vi "TestRingdownEvent.vi"() -> ()   [LabVIEW 2014, in "EventModule.lvlib"]
uses:
  EventModule.lvlib
  EventPlugins/EventPluginBaseClass/TypeDefs/clEvtConfig.ctl
  PublicAPI/Arguments/Requests/dblEvtParams.ctl
  PublicAPI/Arguments/Requests/dblTimeArray.ctl
  EventPlugins/EventPluginBaseClass/TypeDefs/clEvtReportArray.ctl
  EventPlugins/EventPluginBaseClass/TypeDefs/clEvtReport.ctl
  EventPlugins/EventPluginBaseClass/TypeDefs/dblEvtSignalArray.ctl
  TestInfo.ctl
  <userlib>/NIST/ModuleAdminLib/ModuleAdmin/ModuleAdmin.lvclass
  PublicAPI/Arguments/Broadcasts/clDidInit.ctl
  <userlib>/NIST/ModuleAdminLib/ModuleAdmin/ModuleAdmin.lvclass/ModuleAdmin.ctl
  PublicAPI/Arguments/Requests/clStopArgument.ctl
  PublicAPI/Arguments/Broadcasts/clStatUpdate.ctl
  PublicAPI/Arguments/Broadcasts/clErrorRpt.ctl
  <userlib>/NIST/ModuleAdminLib/ModuleAdmin/Accessors/Read CloneRegRef.vi
  <vilib>/Analysis/1siggen.llb/Ramp Pattern by Delta.vi
  <userlib>/NIST/ModuleAdminLib/CloneRegistration/CloneRegistration.lvclass
  EventPlugins/EventPluginBaseClass/EventPluginBaseClass.lvclass
  <vilib>/Analysis/NI_AALBase.lvlib
panel:
  in  "End Time":dbl=10.0
  in  "Start Time":dbl
  in  "Plugin Type":u16(ring)=3 items=["C37.118.1", "Event From CSV", "IEEEBusSystem", "Ringdown", "60255Harm", "User1", "User2"]
  in  "btnGetEvtSignal":bool
  out "dblEventSignalArray":T1
  out "PathToPluginIniFileReport":path=path "P:/Framework/Events/EventPlugins/SSEvtPlugin/SteadyStateEventPlugin.ini"
  in  "btnReadPathToPlugin":bool
  in  "btnGetEvtReportArray":bool
  out "clEvtReportArray":T2 {"Synx" format="%#_4g"}
  in  "btnReadEvtParams":bool
  in  "btnWriteEvtParams":bool
  in  "btnReadTimeArray":bool
  in  "btnWriteTimeArray":bool
  out "dblTimeArrayReport":T4
  out "dblEvtParamsReport":T5
  out "dblTimeArray":T4=[0.0, 0.05, 0.1, 0.15000000000000002, 0.2]
  in  "dblEvtParams":T5=[[0.0, 0.34657, 0.69677, 1.297, 1.4569, 6.0606, 7.2288, 8.9506, 11.705, 18.574], [1000.0, 24.879, 55.751, 46.204, 36.867, 1.995, 0.82578, 1.5487, 1.8652, 1.6268], [0.0, 1.876, 0.28983, 1.5993, 2.6728, 3.9286, 1.2558, 3.3379, 3.6506, 7.1708], [0.0, -67.696, -60.912, 99.138, -123.76, 176.38, -149.46, -106.27, -18.535, -59.29], [0.0, 0.0, 0.58767, 0.6985, 1.3263, 2.7275, 7.1783, 8.122, 14.704, 15.622], [200.0, 31.231, 41.605, 48.38, 1.6511, 0.84175, 2.671, 0.64619, 0.78365, 0.6061], [0.0, 6.2405, 2.3071, 0.28998, 1.025, 3.6069, 15.284, 3.3041, 2.4034, 2.5242], [0.0, 180.0, 37.683, 113.63, 41.526, 4.7072, 5.0124, -177.41, -50.759, 41.697], [568.0, 0.0, 0.0, 0.0, 0.0, 0.0, 0.0, 0.0, 0.0, 0.0], [0.0, 0.0, 0.0, 0.0, 0.0, 0.0, 0.0, 0.0, 0.0, 0.0], [0.0, 0.0, 0.0, 0.0, 0.0, 0.0, 0.0, 0.0, 0.0, 0.0], [0.0, 0.0, 0.0, 0.0, 0.0, 0.0, 0.0, 0.0, 0.0, 0.0], [0.0, 0.0, 0.0, 0.0, 0.0, 0.0, 0.0, 0.0, 0.0, 0.0]]
  out "clEvtConfigReport":T6={"T0(UTC)"=0.0, "F0"=0.0, "Fs"=60, "FSamp"=0, "bPosSeq"=FALSE}
  in  "btnReadEvtConfig":bool
  in  "clEvtConfig":T6={"T0(UTC)"=0.0, "F0"=60.0, "Fs"=60, "FSamp"=960, "bPosSeq"=FALSE}
  in  "btnWriteEvtConfig":bool
  in  "btnLoadPlugin":bool
  in  "btnRemove":bool
  out "Status Log":string
  out "Active Modules (Array)":string[](array[string])
  in  "btnAdd":bool
  in  "btnStop":bool
  in  "Select Module":i32(ring)=-1 caption="Select Module to send Request" items=["All"=-1, "4140002"=4140002]
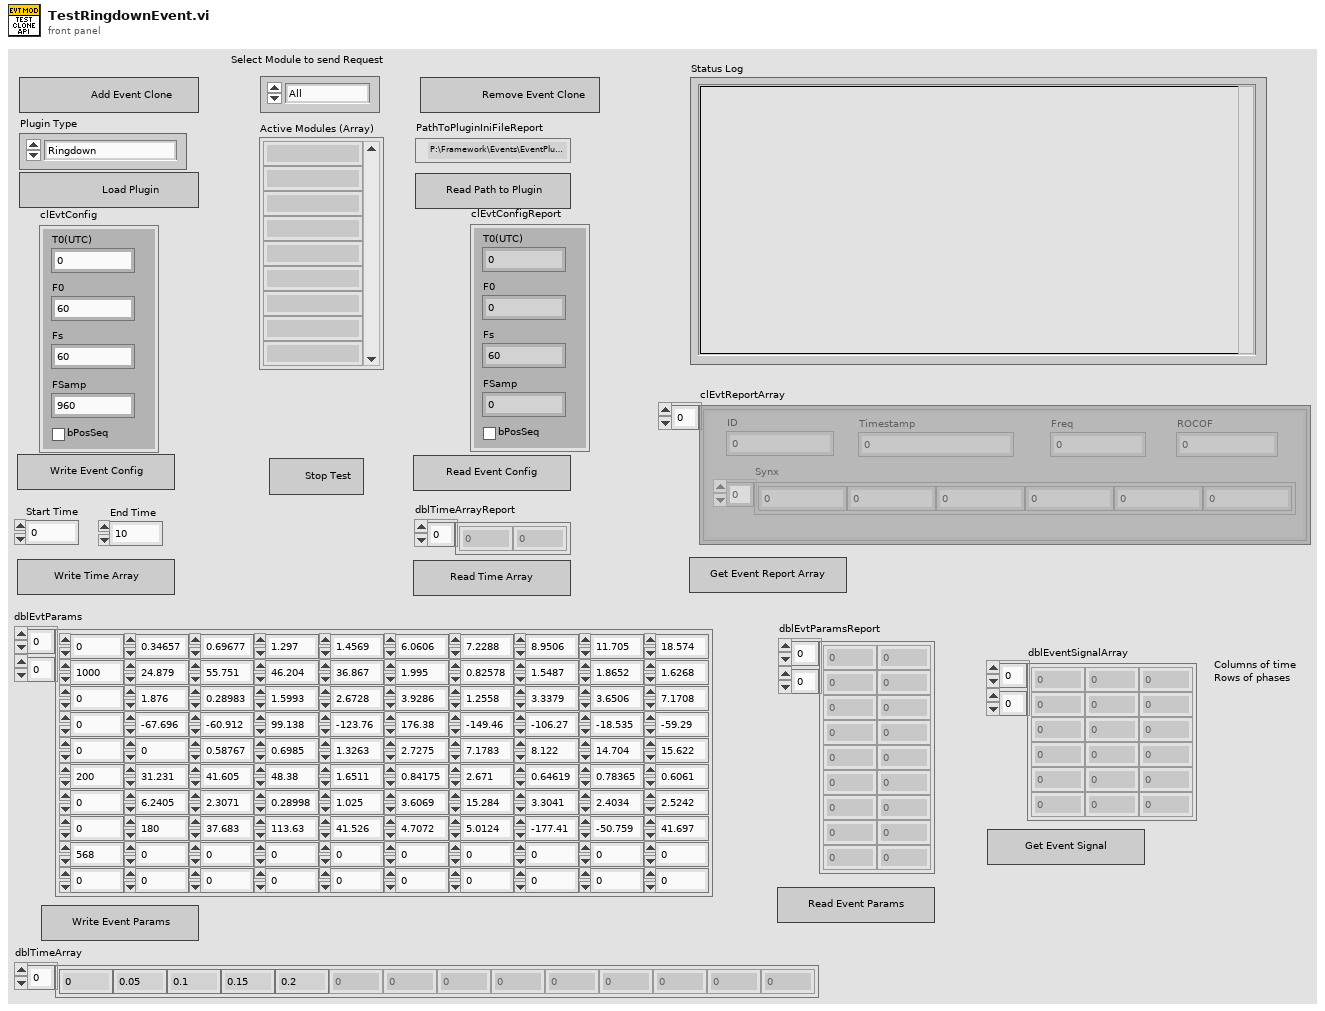
[diagram p1: front panel]
types:
  T1 = typedef "EventPlugins.lvlib/EventPluginBaseClass.lvclass/dblEvtSignalArray.ctl" = dbl[][]
  T2 = typedef "EventPlugins.lvlib/EventPluginBaseClass.lvclass/clEvtReportArray.ctl" = T3[]
  T3 = typedef "EventPlugins.lvlib/EventPluginBaseClass.lvclass/clEvtReport.ctl" = cluster{"Timestamp":dbl, "Synx":cdb[], "Freq":dbl, "ROCOF":dbl, "ID":i16}
  T4 = typedef "EventModule.lvlib/dblTimeArray.ctl" = dbl[]
  T5 = typedef "EventModule.lvlib/dblEvtParams.ctl" = dbl[][]
  T6 = typedef "EventPlugins.lvlib/EventPluginBaseClass.lvclass/clEvtConfig.ctl" = cluster{"T0(UTC)":dbl, "F0":dbl, "Fs":i32, "FSamp":u32, "bPosSeq":bool}
  T7 = typedef "EventModule.lvlib/TestInfo.ctl" = cluster{"PluginIniFilePaths":path[]}
  T8 = typedef "EventModule.lvlib/clBroadcastEvents.ctl" = cluster{"DidInit":refnum<user-event>, "StatusUpdate":refnum<user-event>, "ErrorReport":refnum<user-event>, "DidStop":refnum<user-event>, "ReadEvtConfig":refnum<user-event>, "ReadTimeArray":refnum<user-event>, "ReadEvtParams":refnum<user-event>, "GetEvtReportArray":refnum<user-event>, "ReadPathToPlugin":refnum<user-event>, "GetEvtSignal":refnum<user-event>, "ReadBusNumber":refnum<user-event>}
  T9 = typedef "EventModule.lvlib/clDidInit.ctl" = cluster{"Init?":bool, "ModuleAdmin":refnum<class "ModuleAdmin.lvclass">}
  T10 = typedef "EventModule.lvlib/clStopArgument.ctl" = cluster{"Exit via Stop Module Req?":bool, "Wait for Module to stop?":bool, "ModuleAdmin":refnum<class "ModuleAdmin.lvclass">}
  T11 = typedef "EventModule.lvlib/clStatUpdate.ctl" = cluster{"Status":string}
  T12 = typedef "EventModule.lvlib/clErrorRpt.ctl" = cluster{"error":errorcluster, "AdditionalInfo":string}
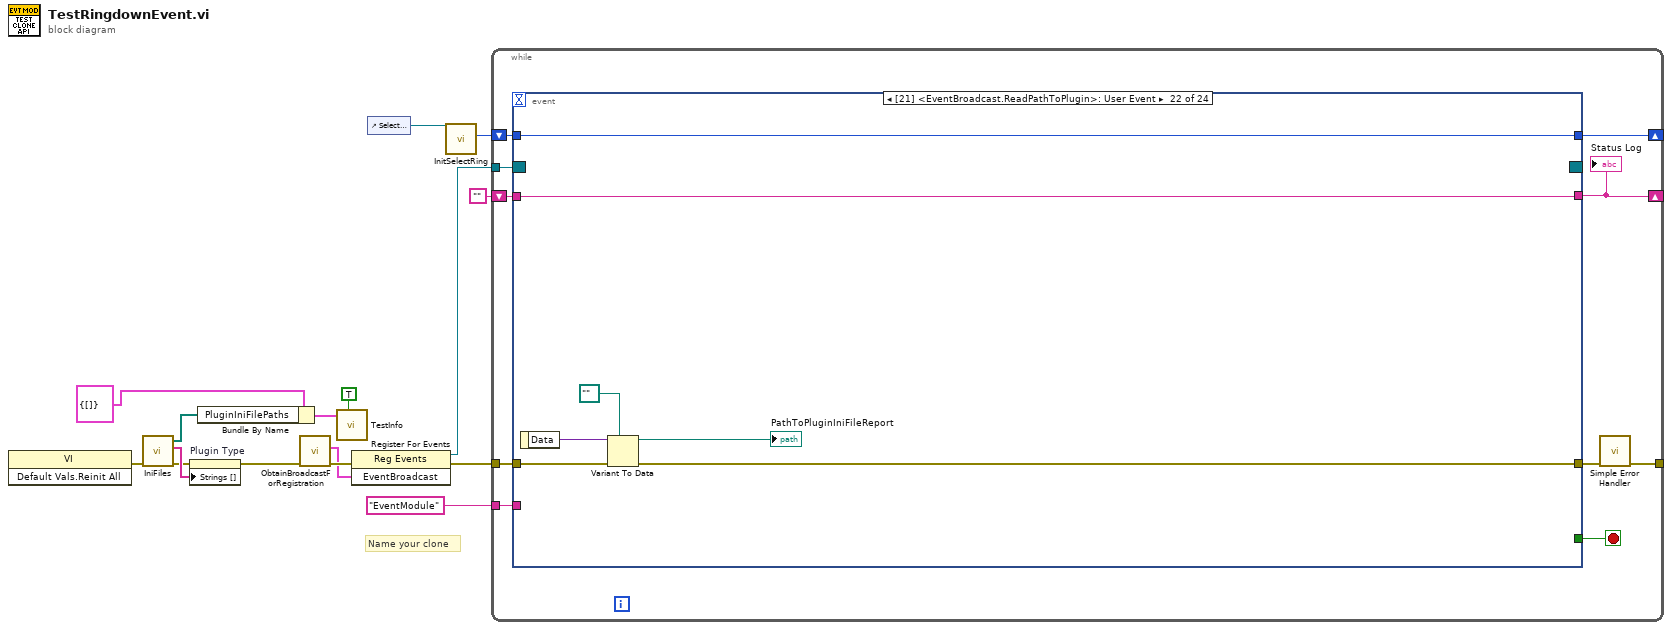
[diagram p0: block diagram]
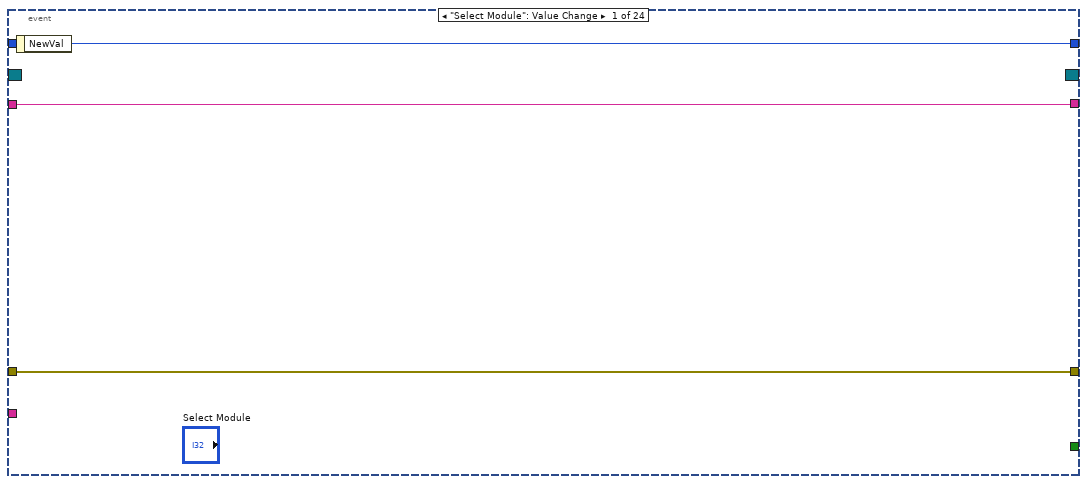
[diagram p2: hidden frame]
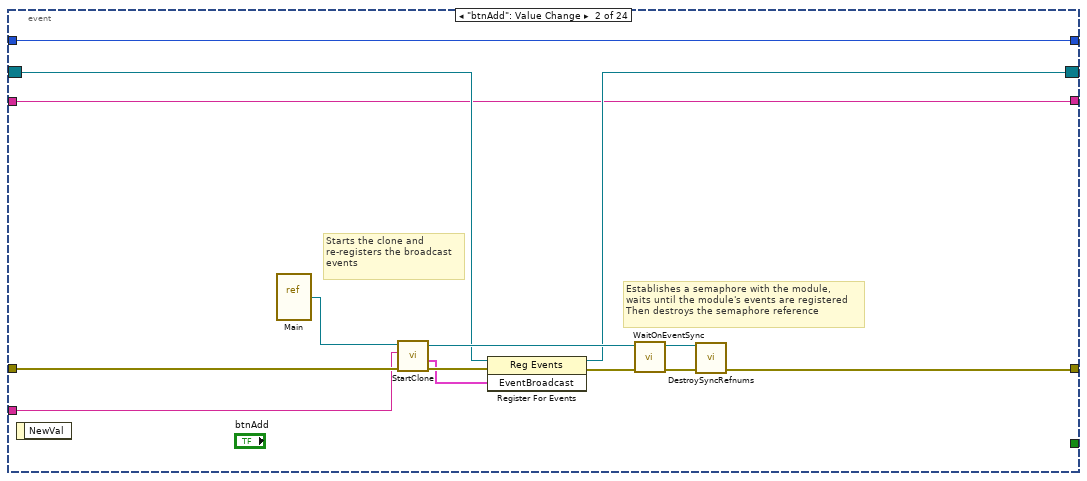
[diagram p3: hidden frame]
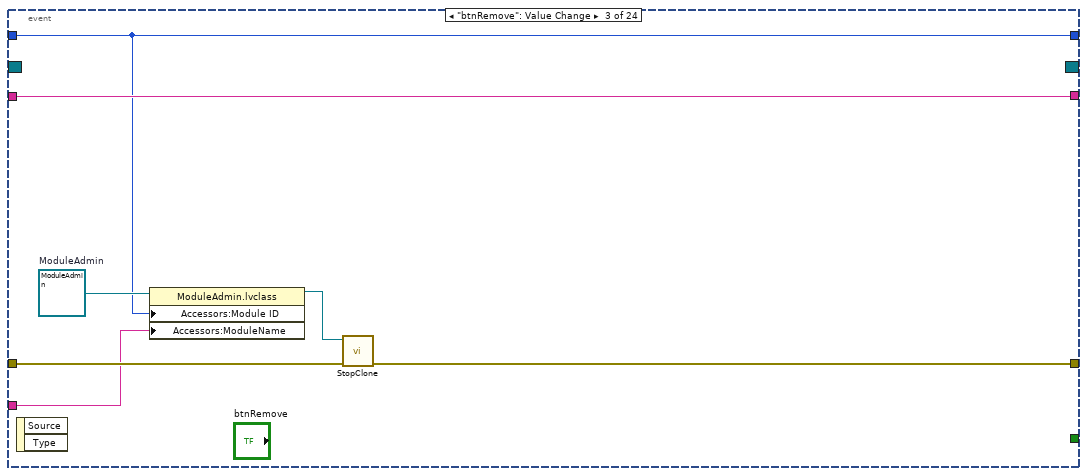
[diagram p4: hidden frame]
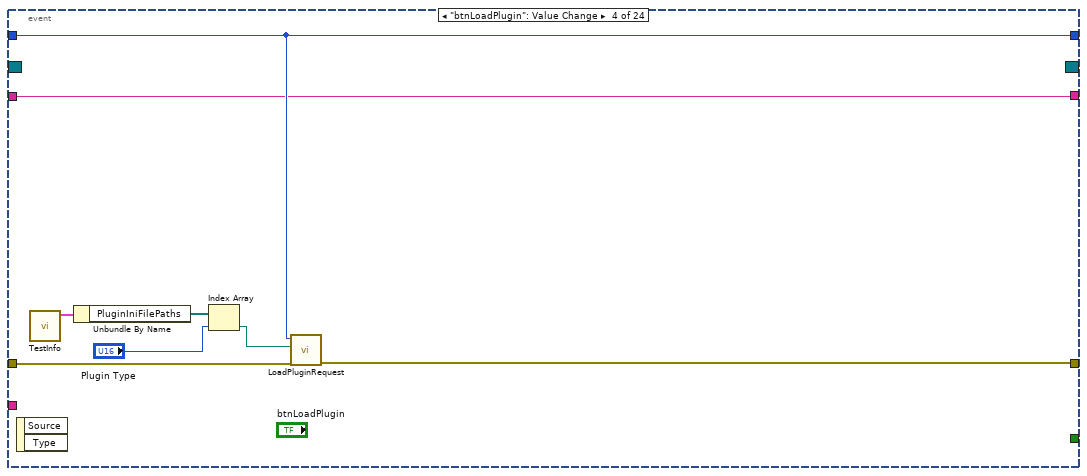
[diagram p5: hidden frame]
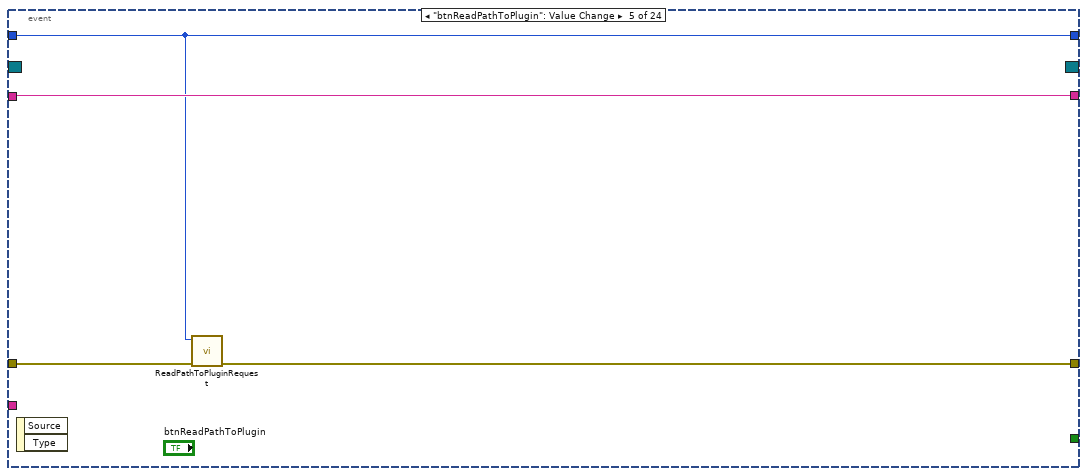
[diagram p6: hidden frame]
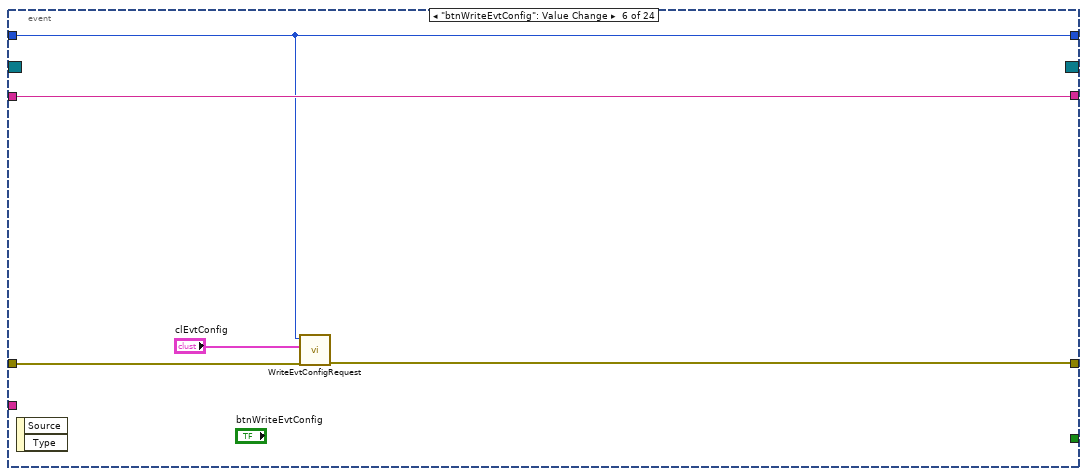
[diagram p7: hidden frame]
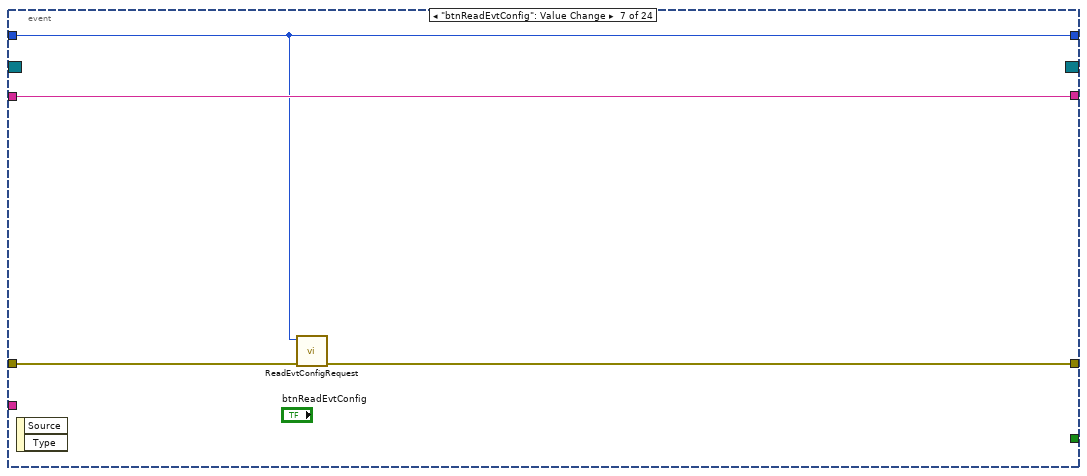
[diagram p8: hidden frame]
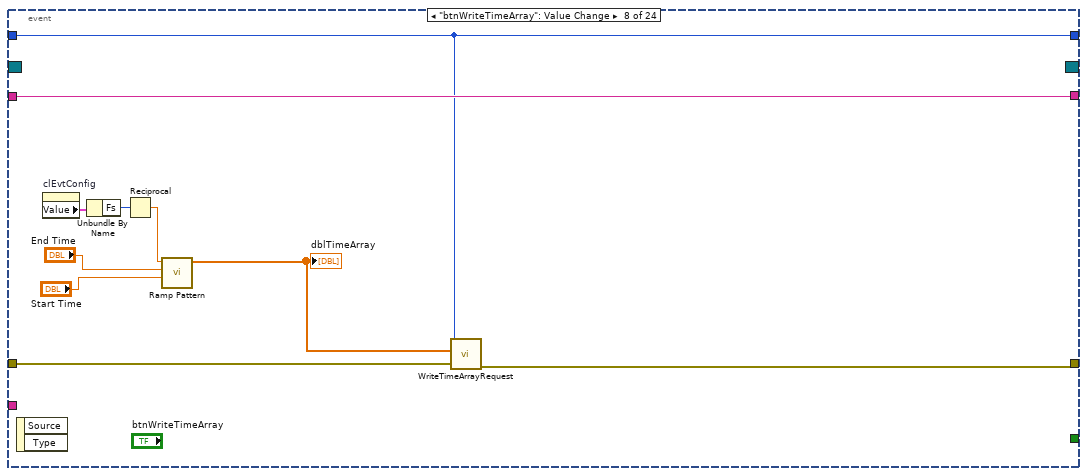
[diagram p9: hidden frame]
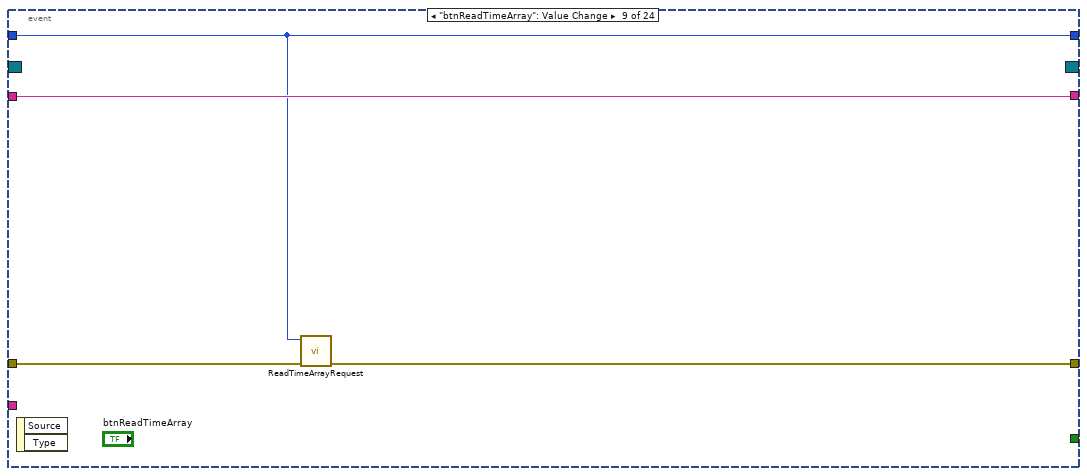
[diagram p10: hidden frame]
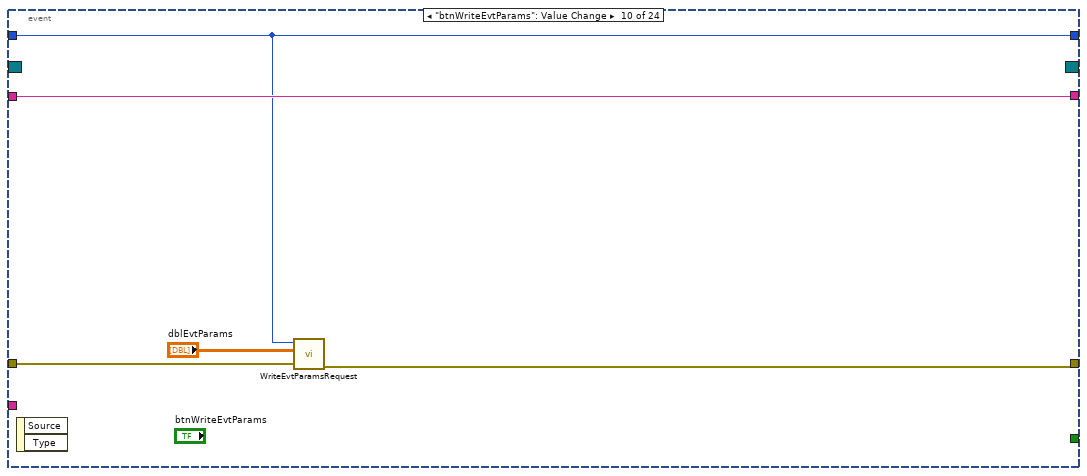
[diagram p11: hidden frame]
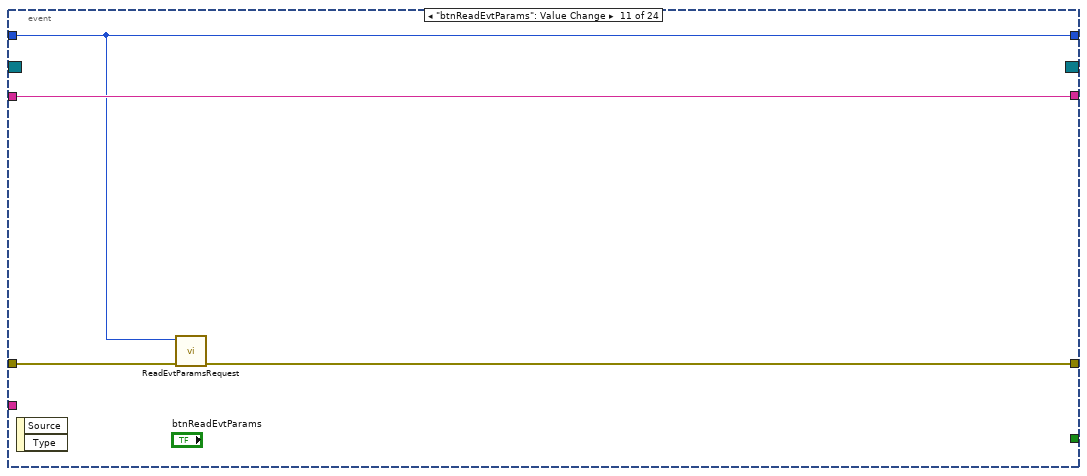
[diagram p12: hidden frame]
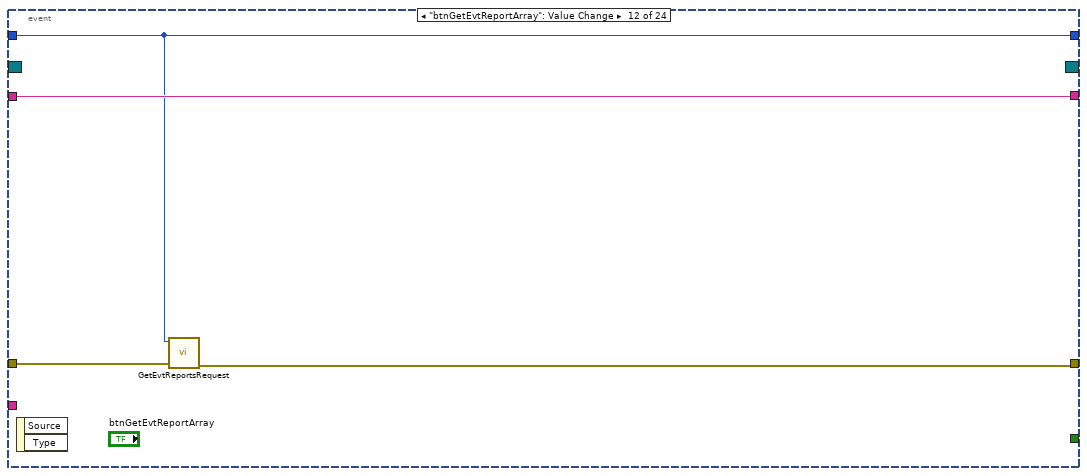
[diagram p13: hidden frame]
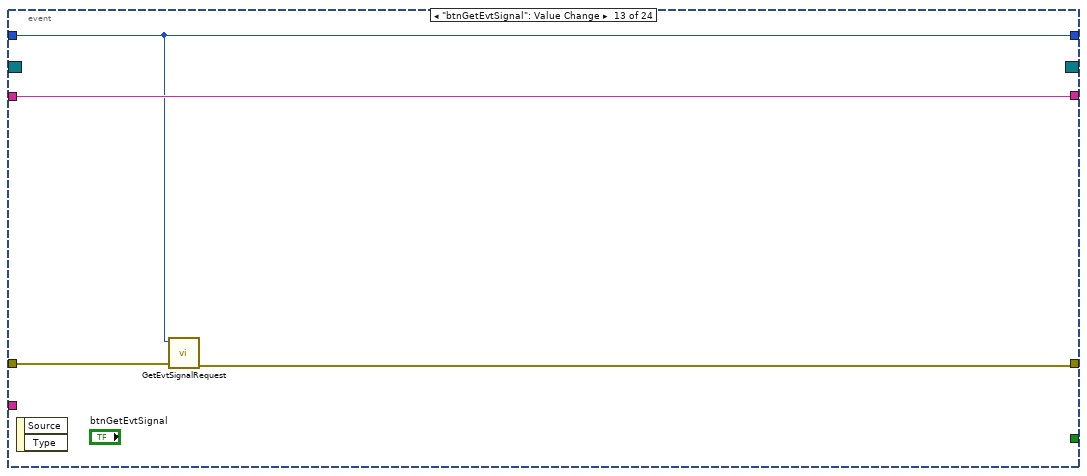
[diagram p14: hidden frame]
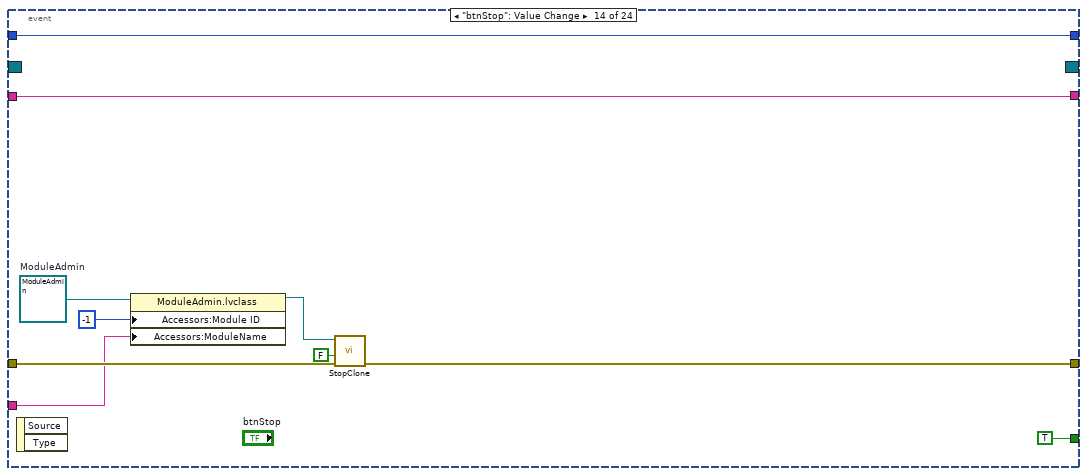
[diagram p15: hidden frame]
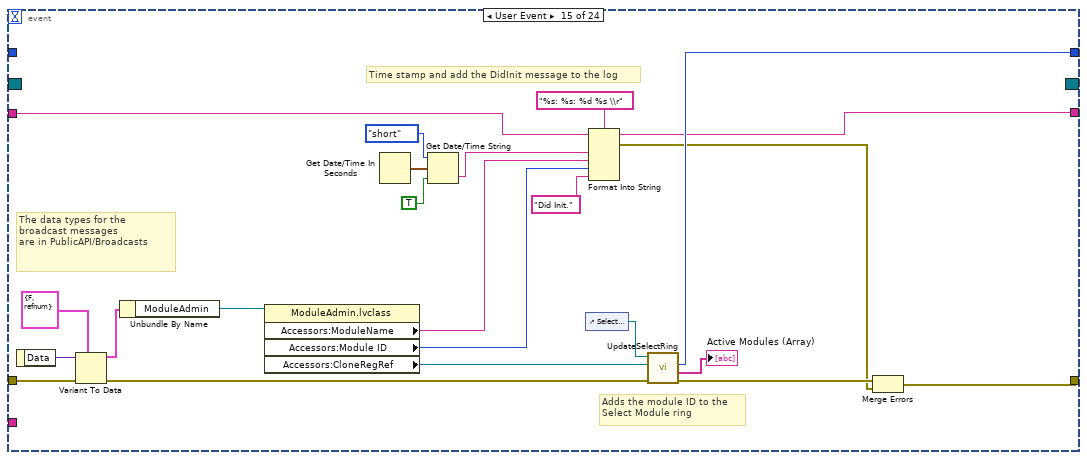
[diagram p16: hidden frame]
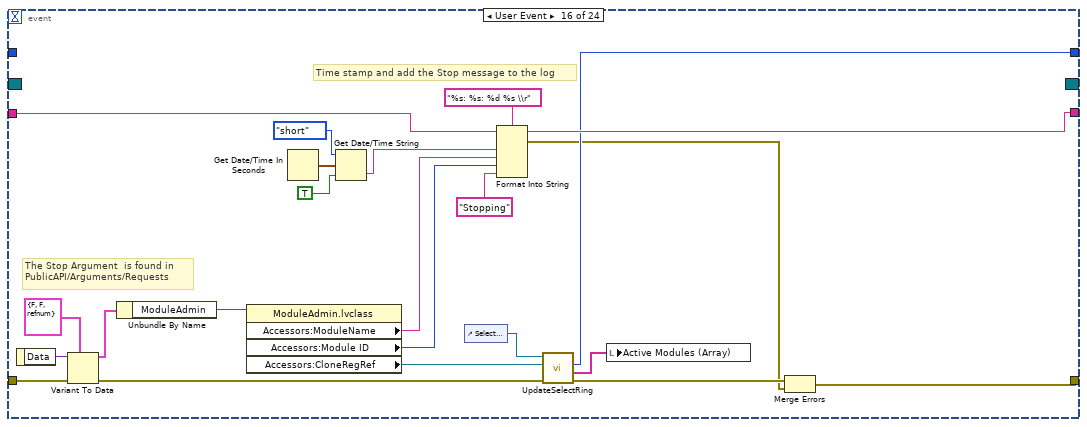
[diagram p17: hidden frame]
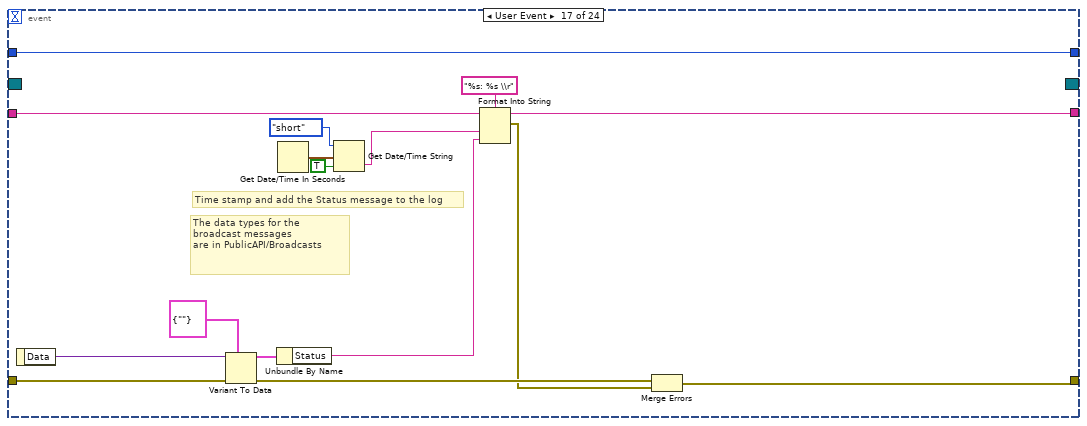
[diagram p18: hidden frame]
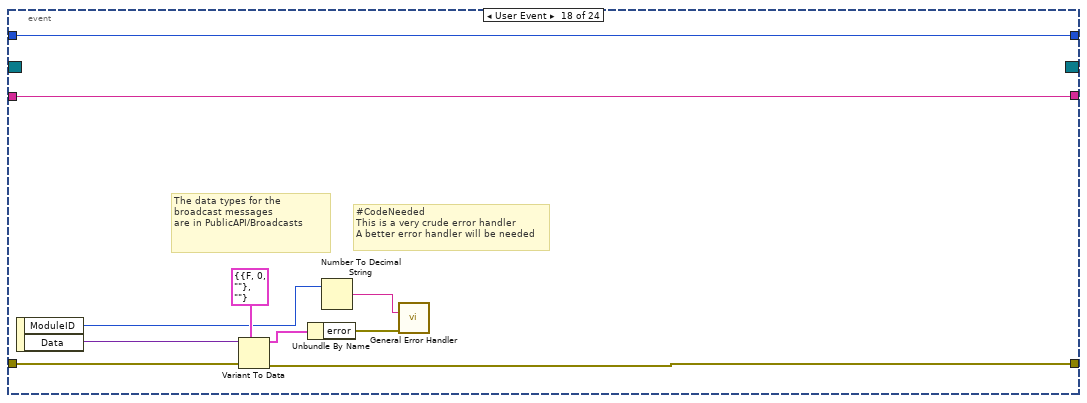
[diagram p19: hidden frame]
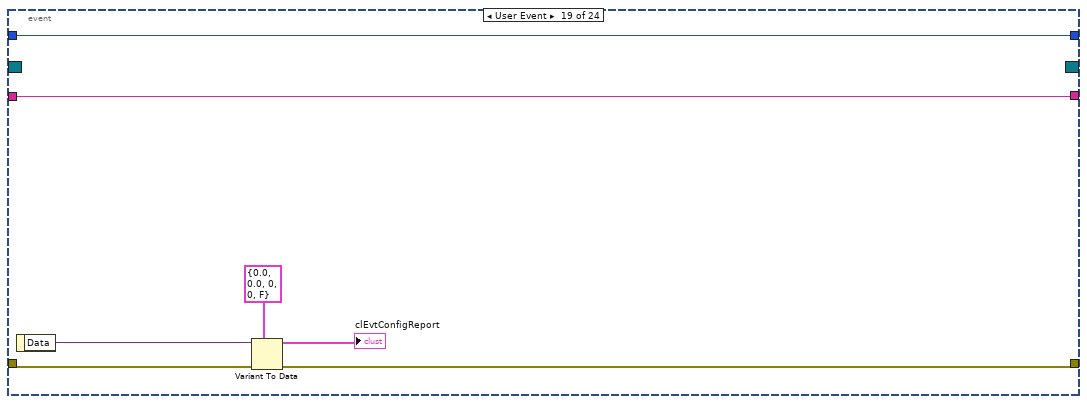
[diagram p20: hidden frame]
diagram:
  # "Name your clone"
  n1 = invoke class="VI" method="Default Vals.Reinit All"() -> (error out=w8:errorcluster)  [unwired: 3 in, 2 out]
  n2 = call "IniFiles.vi"("error in"=w8) -> ("error out"=w6:errorcluster, "Types"=w7:string[], "IniFilePaths"=w3:path[])  [unwired: 8 in]
  n3 = property on="Plugin Type" class="Ring (strict)"(error in=w6, "Strings []"=w7) -> (error out=w5:errorcluster)  [unwired: 1 in, 1 out]
  n4 = Bundle By Name(cluster=T7 {"PluginIniFilePaths"=[]} ("TestInfo"), "PluginIniFilePaths"=w3) -> (w2:T7)
  n5 = call "ObtainBroadcastForRegistration.vi"("error in (no error)"=w5) -> ("error out"=w14:errorcluster, "EventBroadcast"=w13:T8)  [unwired: 9 in]
  n6 = call "TestInfo.vi"("Set (f)"=TRUE, "TestInfo"=w2) -> ()  [unwired: 9 in, 1 out]
  n7 = register-events(error in=w14, w13) -> (reference out=w11:refnum<event-registration>, error out=w12:errorcluster)  [unwired: 1 in]
  n8 = control-ref of="Select Module"() -> (w16:refnum<vi>)
  n9 = call "InitSelectRing.vi"("Ring Refnum"=w16) -> ("Module Ring Value"=w15:i32)  [unwired: 9 in, 1 out]
  n10 = while {
    shift-right: [w25] -> _
    shift-left: w15 -> [w26]
    tunnel: w12 -> [w23]
    tunnel: w11 -> [w20]
    tunnel: [w21] -> _
    shift-right: [w19] -> _
    shift-left: "" -> [w18]
    tunnel: "EventModule" ("ModuleName") -> [w17]
    stop <- w24 stop-if-true
    n11 = event shown="[21] <EventBroadcast.ReadPathToPlugin>: User Event" {
      selector: w20 -> [_ w34 _ _ _ _ _ _ _ _ _ _ _ _ _ _ _ _ _ _ _ _ _ _]
      dyn-events: [_ w33 _ _ _ _ _ _ _ _ _ _ _ _ _ _ _ _ _ _ _ _ _ _] -> _
      timeout: _ -> [_ _ _ _ _ _ _ _ _ _ _ _ _ _ _ _ _ _ _ _ _ _ _ _]
      tunnel: w26 -> [_ w43 w45 w57 w59 w64 w68 w78 w84 w87 w92 w95 w99 w112 _ _ w174 w176 w185 w193 w200 w207 w214 w222]
      tunnel: [w29 w43 w45 w57 w59 w64 w68 w78 w84 w87 w92 w95 w99 w112 w130 w145 w174 w176 w185 w193 w200 w207 w214 w222] -> w25
      tunnel: [_ _ _ _ _ _ _ _ _ _ _ _ _ TRUE _ _ _ _ _ _ _ _ _ _] -> w24
      tunnel: w23 -> [w27 w42 w49 w58 w61 w66 w70 w81 w83 w90 w93 w98 w102 w110 w135 w154 w171 w183 w188 w198 w202 w211 w219 w226]
      tunnel: [w27 w35 w48 w56 w60 w63 w69 w80 w82 w88 w91 w97 w101 w108 w118 w142 w162 w182 w187 w197 w203 w209 w218 w225] -> w22
      tunnel: [w28 w31 w50 w55 w62 w67 w71 w79 w85 w89 w94 w96 w100 w107 w122 w151 w165 w175 w186 w192 w201 w208 w215 w223] -> w19
      tunnel: w18 -> [w28 w31 w50 w55 w62 w67 w71 w79 w85 w89 w94 w96 w100 w107 w121 w152 w173 w175 w186 w192 w201 w208 w215 w223]
      tunnel: w17 -> [_ w30 w46 _ _ _ _ _ _ _ _ _ _ w104 _ _ _ _ _ _ _ _ _ _]
      event "Select Module": Value Change {
        n12 = event-data() -> ("NewVal"=w29:i32)  [unwired: 1 in]
      }
      event "btnAdd": Value Change {
        # "Establishes a semaphore with the module,\nwaits until the module's events are registered\nThen destroys the semaphore reference"
        # "Starts the clone and\nre-registers the broadcast \nevents"
        n13 = event-data() -> ()  [unwired: 1 in, 1 out]
        n14 = vi-ref "Main.vi"() -> (w32:refnum<vi>)
        n15 = call "StartClone.vi"("error in (no error)"=w42, "ModuleName"=w30, "VI Refnum"=w32) -> ("error out"=w41:errorcluster, "clBroadcastEvents"=w36:T8, "ModuleAdmin"=w38:refnum<class "ModuleAdmin.lvclass">)  [unwired: 6 in]
        n16 = register-events(reference=w34, error in=w41, w36) -> (reference out=w33:refnum<event-registration>, error out=w40:errorcluster)
        n17 = call <userlib>:"WaitOnEventSync.vi"("error in (no error)"=w40, "ModuleAdmin"=w38) -> ("error out"=w39:errorcluster, "ModuleAdmin"=w37:refnum<class "ModuleAdmin.lvclass">)  [unwired: 8 in]
        n18 = call <userlib>:"DestroySyncRefnums.vi"("error in (no error)"=w39, "ModuleAdmin"=w37) -> ("error out"=w35:errorcluster)  [unwired: 9 in]
      }
      event "btnRemove": Value Change {
        w47 = refnum<class "ModuleAdmin.lvclass"> refnum  # ModuleAdmin
        n19 = event-data() -> ()  [unwired: 1 in, 2 out]
        n20 = property class="ModuleAdmin.lvclass"(reference=w47, "Accessors:Module ID"=w45, "Accessors:ModuleName"=w46) -> (reference out=w44:refnum<class "ModuleAdmin.lvclass">)  [unwired: 1 in, 1 out]
        n21 = call "StopClone.vi"("error in (no error)"=w49, "ModuleAdmin"=w44) -> ("error out"=w48:errorcluster)  [unwired: 9 in]
      }
      event "btnLoadPlugin": Value Change {
        n22 = event-data() -> ()  [unwired: 1 in, 2 out]
        n23 = call "TestInfo.vi"() -> ("TestInfo"=w54:T7)  [unwired: 11 in]
        n24 = Unbundle By Name(w54) -> ("PluginIniFilePaths"=w53:path[])
        n25 = Index Array(array=w53, index="Plugin Type") -> (element=w51:path)
        n26 = call "LoadPluginRequest.vi"("error in (no error)"=w58, "PathToPlugin"=w51, "ModuleID"=w57) -> ("error out"=w56:errorcluster)  [unwired: 8 in]
      }
      event "btnReadPathToPlugin": Value Change {
        n27 = event-data() -> ()  [unwired: 1 in, 2 out]
        n28 = call "ReadPathToPluginRequest.vi"("error in (no error)"=w61, "ModuleID"=w59) -> ("error out"=w60:errorcluster)  [unwired: 9 in]
      }
      event "btnWriteEvtConfig": Value Change {
        n29 = event-data() -> ()  [unwired: 1 in, 2 out]
        n30 = call "WriteEvtConfigRequest.vi"("error in (no error)"=w66, "clEvtConfig"="clEvtConfig", "ModuleID"=w64) -> ("error out"=w63:errorcluster)  [unwired: 8 in]
      }
      event "btnReadEvtConfig": Value Change {
        n31 = event-data() -> ()  [unwired: 1 in, 2 out]
        n32 = call "ReadEvtConfigRequest.vi"("error in (no error)"=w70, "ModuleID"=w68) -> ("error out"=w69:errorcluster)  [unwired: 9 in]
      }
      event "btnWriteTimeArray": Value Change {
        n33 = event-data() -> ()  [unwired: 1 in, 2 out]
        n34 = property on="clEvtConfig" class="Clust (strict)"() -> ("Value"=w75:T6)  [unwired: 2 in, 2 out]
        n35 = Unbundle By Name(w75) -> ("Fs"=w74:i32)
        n36 = Reciprocal(x=w74) -> (1/x=w73:dbl)
        n37 = call-poly <vilib>:"Ramp Pattern.vi"("start"="Start Time", "end"="End Time", "delta"=w73) -> ("Ramp Pattern"=w72:dbl[])  [unwired: 6 in, 2 out]
        "dblTimeArray" <- w72
        n38 = call "WriteTimeArrayRequest.vi"("error in (no error)"=w81, "TimeArray"=w72, "ModuleID"=w78) -> ("error out"=w80:errorcluster)  [unwired: 8 in]
      }
      event "btnReadTimeArray": Value Change {
        n39 = event-data() -> ()  [unwired: 1 in, 2 out]
        n40 = call "ReadTimeArrayRequest.vi"("error in (no error)"=w83, "ModuleID"=w84) -> ("error out"=w82:errorcluster)  [unwired: 9 in]
      }
      event "btnWriteEvtParams": Value Change {
        n41 = event-data() -> ()  [unwired: 1 in, 2 out]
        n42 = call "WriteEvtParamsRequest.vi"("error in (no error)"=w90, "EvtParams"="dblEvtParams", "ModuleID"=w87) -> ("error out"=w88:errorcluster)  [unwired: 8 in]
      }
      event "btnReadEvtParams": Value Change {
        n43 = event-data() -> ()  [unwired: 1 in, 2 out]
        n44 = call "ReadEvtParamsRequest.vi"("error in (no error)"=w93, "ModuleID"=w92) -> ("error out"=w91:errorcluster)  [unwired: 9 in]
      }
      event "btnGetEvtReportArray": Value Change {
        n45 = event-data() -> ()  [unwired: 1 in, 2 out]
        n46 = call "GetEvtReportsRequest.vi"("error in (no error)"=w98, "ModuleID"=w95) -> ("error out"=w97:errorcluster)  [unwired: 9 in]
      }
      event "btnGetEvtSignal": Value Change {
        n47 = event-data() -> ()  [unwired: 1 in, 2 out]
        n48 = call "GetEvtSignalRequest.vi"("error in (no error)"=w102, "ModuleID"=w99) -> ("error out"=w101:errorcluster)  [unwired: 9 in]
      }
      event "btnStop": Value Change {
        w106 = refnum<class "ModuleAdmin.lvclass"> refnum  # ModuleAdmin
        n49 = event-data() -> ()  [unwired: 1 in, 2 out]
        n50 = property class="ModuleAdmin.lvclass"(reference=w106, "Accessors:Module ID"=-1 ("Module ID"), "Accessors:ModuleName"=w104) -> (reference out=w103:refnum<class "ModuleAdmin.lvclass">)  [unwired: 1 in, 1 out]
        n51 = call "StopClone.vi"("error in (no error)"=w110, "Wait for Module to stop?"=FALSE, "ModuleAdmin"=w103) -> ("error out"=w108:errorcluster)  [unwired: 8 in]
      }
      event User Event {
        # "Adds the module ID to the \nSelect Module ring"
        # "Time stamp and add the DidInit message to the log"
        # "The data types for the broadcast messages\nare in PublicAPI/Broadcasts"
        n52 = event-data() -> ("Data"=w134:variant)  [unwired: 1 in]
        n53 = Variant To Data(error in=w135, type=T9 {"Init?"=FALSE, "ModuleAdmin"=refnum} ("clDidInit"), Variant=w134) -> (data=w127:T9, error out=w132:errorcluster)
        n54 = Unbundle By Name(w127) -> ("ModuleAdmin"=w126:refnum<class "ModuleAdmin.lvclass">)
        n55 = property class="ModuleAdmin.lvclass"(reference=w126) -> ("Accessors:ModuleName"=w115:string, "Accessors:Module ID"=w114:i32, "Accessors:CloneRegRef"=w113:refnum<data-value>)  [unwired: 1 in, 2 out]
        n56 = Get Date/Time In Seconds() -> (seconds since 1Jan1904=w124:timestamp)
        n57 = Get Date/Time String(date format (0)=enum16{"short", "long", "abbreviated"}."short", seconds (now)=w124, want seconds? (F)=TRUE) -> (time string=w128:string)  [unwired: 1 out]
        n58 = control-ref of="Select Module"() -> (w131:refnum<vi>)
        n59 = Format Into String(format string="%s: %s: %d %s \\r", initial string=w121, w128, w115, w114, "Did Init.") -> (resulting string=w122:string, error out=w119:errorcluster)  [unwired: 1 in]
        n60 = call "UpdateSelectRing.vi"("error in (no error)"=w132, "CloneRegRef"=w113, "Ring Refnum"=w131) -> ("error out"=w120:errorcluster, "ActiveModules"=→"Active Modules (Array)":string[], "Module Ring Value"=w130:i32)  [unwired: 6 in]
        n61 = Merge Errors(w120, w119) -> (w118:errorcluster)
      }
      event User Event {
        # "Time stamp and add the Stop message to the log"
        # "The Stop Argument  is found in\nPublicAPI/Arguments/Requests"
        n62 = event-data() -> ("Data"=w153:variant)  [unwired: 1 in]
        n63 = Variant To Data(error in=w154, type=T10 {"Exit via Stop Module Req?"=FALSE, "Wait for Module to stop?"=FALSE, "ModuleAdmin"=refnum} ("Stop Argument"), Variant=w153) -> (data=w149:T10, error out=w148:errorcluster)
        n64 = Unbundle By Name(w149) -> ("ModuleAdmin"=w140:refnum<class "ModuleAdmin.lvclass">)
        n65 = property class="ModuleAdmin.lvclass"(reference=w140) -> ("Accessors:ModuleName"=w137:string, "Accessors:Module ID"=w136:i32, "Accessors:CloneRegRef"=w139:refnum<data-value>)  [unwired: 1 in, 2 out]
        n66 = Get Date/Time In Seconds() -> (seconds since 1Jan1904=w156:timestamp)
        n67 = Get Date/Time String(date format (0)=enum16{"short", "long", "abbreviated"}."short", seconds (now)=w156, want seconds? (F)=TRUE) -> (time string=w158:string)  [unwired: 1 out]
        n68 = control-ref of="Select Module"() -> (w147:refnum<vi>)
        n69 = Format Into String(format string="%s: %s: %d %s \\r", initial string=w152, w158, w137, w136, "Stopping") -> (resulting string=w151:string, error out=w143:errorcluster)  [unwired: 1 in]
        n70 = call "UpdateSelectRing.vi"("error in (no error)"=w148, "CloneRegRef"=w139, "Ring Refnum"=w147) -> ("error out"=w144:errorcluster, "ActiveModules"=w146:string[], "Module Ring Value"=w145:i32)  [unwired: 6 in]
        n71 = local write "Active Modules (Array)"(w146) -> ()
        n72 = Merge Errors(w144, w143) -> (w142:errorcluster)
      }
      event User Event {
        # "Time stamp and add the Status message to the log"
        # "The data types for the broadcast messages\nare in PublicAPI/Broadcasts"
        n73 = event-data() -> ("Data"=w170:variant)  [unwired: 1 in]
        n74 = Variant To Data(error in=w171, type=T11 {"Status"=""} ("clStatUpdate"), Variant=w170) -> (data=w168:T11, error out=w164:errorcluster)
        n75 = Unbundle By Name(w168) -> ("Status"=w166:string)
        n76 = Get Date/Time In Seconds() -> (seconds since 1Jan1904=w167:timestamp)
        n77 = Get Date/Time String(date format (0)=enum16{"short", "long", "abbreviated"}."short", seconds (now)=w167, want seconds? (F)=TRUE) -> (time string=w159:string)  [unwired: 1 out]
        n78 = Format Into String(format string="%s: %s \\r", initial string=w173, w159, w166) -> (resulting string=w165:string, error out=w163:errorcluster)  [unwired: 1 in]
        n79 = Merge Errors(w164, w163) -> (w162:errorcluster)
      }
      event User Event {
        # "#CodeNeeded\nThis is a very crude error handler\nA better error handler will be needed"
        # "The data types for the broadcast messages\nare in PublicAPI/Broadcasts"
        n80 = event-data() -> ("ModuleID"=w179:i32, "Data"=w184:variant)  [unwired: 1 in]
        n81 = Variant To Data(error in=w183, type=T12 {"error"={"status"=FALSE, "code"=0, "source"=""}, "AdditionalInfo"=""} ("Cluster"), Variant=w184) -> (data=w180:T12, error out=w182:errorcluster)
        n82 = Unbundle By Name(w180) -> ("error"=w178:errorcluster)
        n83 = Number To Decimal String(number=w179) -> (decimal integer string=w177:string)  [unwired: 1 in]
        n84 = call <vilib>:"General Error Handler.vi"("[error source] (\" \")"=w177, "error in (no error)"=w178) -> ()  [unwired: 9 in, 5 out]
      }
      event User Event {
        n85 = event-data() -> ("Data"=w191:variant)  [unwired: 1 in]
        n86 = Variant To Data(error in=w188, type=T6 {"T0(UTC)"=0.0, "F0"=0.0, "Fs"=0, "FSamp"=0, "bPosSeq"=FALSE} ("clEvtConfig"), Variant=w191) -> (data=→"clEvtConfigReport":T6, error out=w187:errorcluster)
      }
      event User Event {
        w194 = T4 []  # TimeArray
        n87 = event-data() -> ("Data"=w195:variant)  [unwired: 1 in]
        n88 = Variant To Data(error in=w198, type=w194, Variant=w195) -> (data=→"dblTimeArrayReport":T4, error out=w197:errorcluster)
      }
      event User Event {
        w205 = T5 []  # SignalParams
        n89 = event-data() -> ("Data"=w199:variant)  [unwired: 1 in]
        n90 = Variant To Data(error in=w202, type=w205, Variant=w199) -> (data=→"dblEvtParamsReport":T5, error out=w203:errorcluster)
      }
      event User Event {
        n91 = event-data() -> ("Data"=w212:variant)  [unwired: 1 in]
        n92 = Variant To Data(error in=w211, type=path "", Variant=w212) -> (data=→"PathToPluginIniFileReport":path, error out=w209:errorcluster)
      }
      event User Event {
        w213 = T2 []  # ReportArray
        n93 = event-data() -> ("Data"=w217:variant)  [unwired: 1 in]
        n94 = Variant To Data(error in=w219, type=w213, Variant=w217) -> (data=→"clEvtReportArray":T2, error out=w218:errorcluster)
      }
      event User Event {
        n95 = event-data() -> ("Data"=w224:variant)  [unwired: 1 in]
        n96 = Variant To Data(error in=w226, type=T1 [] ("dblEventSignalArray"), Variant=w224) -> (data=→"dblEventSignalArray":T1, error out=w225:errorcluster)
      }
    }
    "Status Log" <- w19
    n97 = call <vilib>:"Simple Error Handler.vi"("error in (no error)"=w22) -> ("error out"=w21:errorcluster)  [unwired: 4 in, 4 out]
  }
